vi "PH_GUI.set XY graph GUI object.vi"(2 "XY Graph GUI Ref":refnum<vi>, 3 "Value Cluster":cluster{dbl[], dbl[]}, 5 "error in":errorcluster, 7 "Set Full X-Axis (false)":bool, 9 "Set Full Y-Axis (false)":bool) -> (19 "error out":errorcluster)   [LabVIEW 2014, in "PH_Common.lvlib"]
doc: "Sets value and more for the referenced GUI object."
uses:
  PH_Common.lvlib
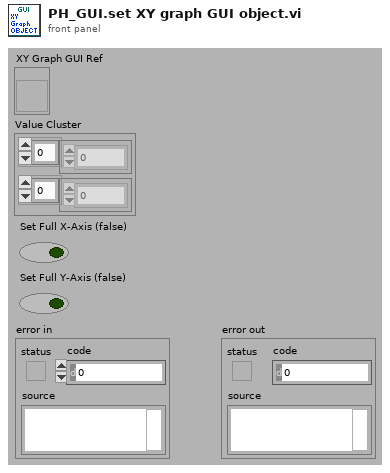
[diagram p1: front panel]
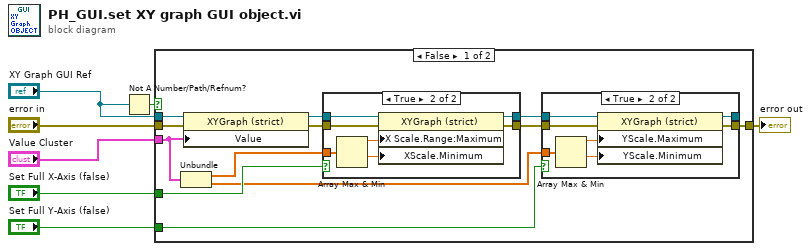
[diagram p0: block diagram]
diagram:
  n1 = Not A Number/Path/Refnum?(number/path/refnum="XY Graph GUI Ref") -> (NaN/Path/Refnum?=w3:bool)
  n2 = case shown="False" w3 {
    tunnel: "error in" -> [w19 w38]
    tunnel: [w10 w38] -> w6
    tunnel: "XY Graph GUI Ref" -> [w18 _]
    tunnel: "Value Cluster" -> [w14 _]
    tunnel: "Set Full X-Axis (false)" -> [w15 _]
    tunnel: "Set Full Y-Axis (false)" -> [w8 _]
    frame False {
      n3 = Unbundle(w14) -> (w13:dbl[], w9:dbl[])
      n4 = property on="Property Node" class="XYGraph (strict)"(reference=w18, error in=w19, "Value"=w14) -> (reference out=w16:refnum<vi>, error out=w17:errorcluster)
      n5 = case shown="True" w15 {
        tunnel: [w29 w37] -> w12
        tunnel: w17 -> [w29 w36]
        tunnel: w16 -> [w30 w35]
        tunnel: [w30 w34] -> w11
        tunnel: w13 -> [_ w33]
        frame False {
        }
        frame True {
          n6 = Array Max & Min(array=w33) -> (max value=w32:dbl, min value=w31:dbl)  [unwired: 2 out]
          n7 = property on="Property Node" class="XYGraph (strict)"(reference=w35, error in=w36, "X Scale.Range:Maximum"=w32, "XScale.Minimum"=w31) -> (reference out=w34:refnum<vi>, error out=w37:errorcluster)
        }
      }
      n8 = case shown="True" w8 {
        tunnel: [w20 w28] -> w10
        tunnel: w12 -> [w20 w27]
        tunnel: w11 -> [w21 w26]
        tunnel: [w21 w25] -> _
        tunnel: w9 -> [_ w24]
        frame False {
        }
        frame True {
          n9 = Array Max & Min(array=w24) -> (max value=w23:dbl, min value=w22:dbl)  [unwired: 2 out]
          n10 = property on="Property Node" class="XYGraph (strict)"(reference=w26, error in=w27, "YScale.Maximum"=w23, "YScale.Minimum"=w22) -> (reference out=w25:refnum<vi>, error out=w28:errorcluster)
        }
      }
    }
    frame True {
    }
  }
  "error out" <- w6
